vi "Spherical Hankel Function hn.vi"(9 "type":i32(ring) items=["First Kind", "Second Kind"], 10 "n":i32, 11 "x":dbl) -> (3 "hn(x)":cdb)   [LabVIEW 2020, in "NI_AAL_MathFunc.lvlib"]
doc: "Computes the spherical Hankel function, which is also known as the spherical Bessel function of the third kind."
uses:
  <vilib>/gmath/NI_AAL_MathFunc.lvlib
  <vilib>/gmath/NI_Gmath.lvlib
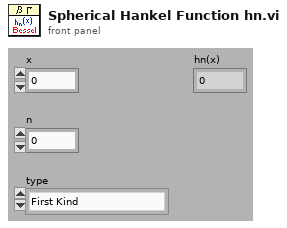
[diagram p1: front panel]
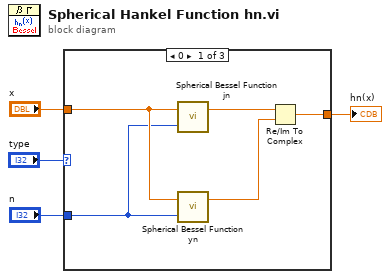
[diagram p0: block diagram]
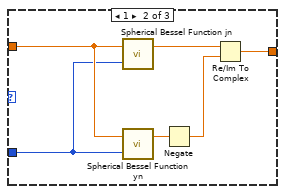
[diagram p2: hidden frame]
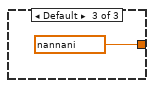
[diagram p3: hidden frame]
diagram:
  n1 = case shown="0" "type" {
    tunnel: "x" -> [w9 w14 _]
    tunnel: "n" -> [w8 w13 _]
    tunnel: [w5 w10 cdb nan+nani ("Hv(x)")] -> w2
    frame 0 {
      n2 = call <vilib>:"Spherical Bessel Function jn.vi"("n"=w8, "x"=w9) -> ("jn(x)"=w7:dbl)  [unwired: 1 in]
      n3 = call <vilib>:"Spherical Bessel Function yn.vi"("n"=w8, "x"=w9) -> ("yn(x)"=w6:dbl)  [unwired: 1 in]
      n4 = Re/Im To Complex(1:w6, 2:w7) -> (0:w5:cdb)
    }
    frame 1 {
      n5 = call <vilib>:"Spherical Bessel Function jn.vi"("n"=w13, "x"=w14) -> ("jn(x)"=w15:dbl)  [unwired: 1 in]
      n6 = call <vilib>:"Spherical Bessel Function yn.vi"("n"=w13, "x"=w14) -> ("yn(x)"=w12:dbl)  [unwired: 1 in]
      n7 = Negate(x=w12) -> (-x=w11:dbl)
      n8 = Re/Im To Complex(1:w11, 2:w15) -> (0:w10:cdb)
    }
    frame Default {
    }
  }
  "hn(x)" <- w2
